vi "1B_TimeIntervals.vi"(0 "appended array":timestamp[](array[timestamp])) -> (1 "Time Intervals":dbl[](array[numeric]), 2 "Time from start":dbl[](array[numeric]))   [LabVIEW 2010]
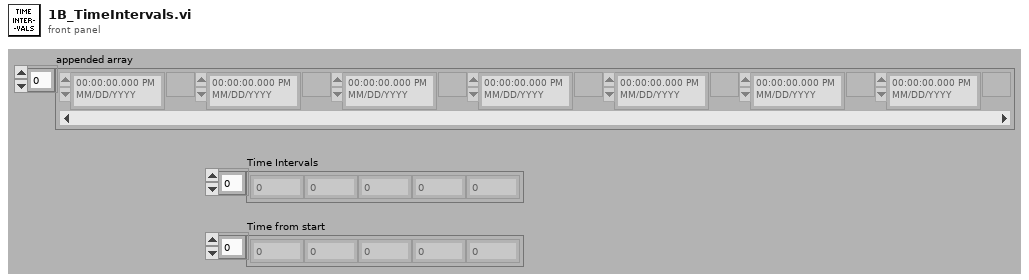
[diagram p1: front panel]
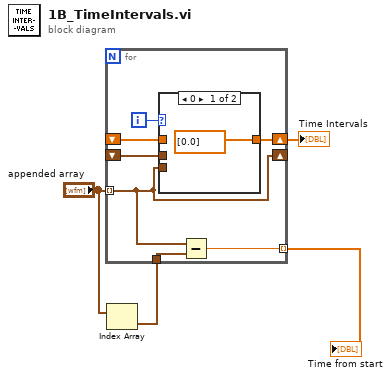
[diagram p0: block diagram]
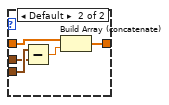
[diagram p2: hidden frame]
diagram:
  n1 = Index Array(array="appended array") -> (element=w2:timestamp)  [unwired: 1 in]
  n2 = for {
    tunnel: "appended array" -> [w7] mode=indexing
    shift-right: [w7] -> _
    shift-left: _ -> [w11]
    shift-right: [w8] -> w4
    shift-left: _ -> [w9]
    tunnel: w2 -> [w6]
    tunnel: [w5] -> w1 mode=indexing
    i -> [w10]
    n3 = case shown="0" w10 {
      tunnel: w7 -> [_ w17]
      tunnel: w11 -> [_ w16]
      tunnel: w9 -> [_ w15]
      tunnel: [dbl[] [0.0] w13] -> w8
      frame 0 {
      }
      frame Default {
        n4 = Subtract(x=w17, y=w16) -> (x-y=w14:dbl)
        n5 = Build Array (concatenate)(w15, w14) -> (w13:dbl[])
      }
    }
    n6 = Subtract(x=w7, y=w6) -> (x-y=w5:dbl)
  }
  "Time Intervals" <- w4
  "Time from start" <- w1
